vi "Read Data.vi"(8 "error in (no error)":errorcluster, 11 "VISA resource name":refnum<visa-resource-name>) -> (0 "error out":errorcluster, 1 "Return String":string, 2 "Data Value":dbl format="%_10f", 3 "VISA resource name out":refnum<visa-resource-name>)   [LabVIEW 2019, in "BK Precision 1823A.lvlib"]
doc: "This VI returns the measured data corresponding to the display of the counter."
uses:
  BK Precision 1823A.lvlib
panel:
  # "Units"
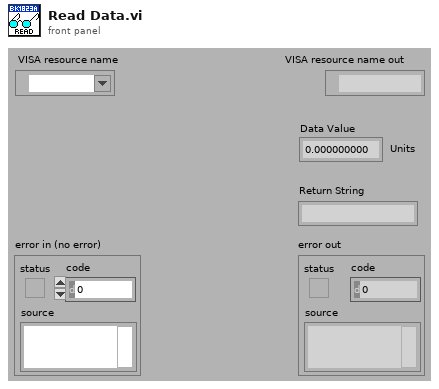
[diagram p1: front panel]
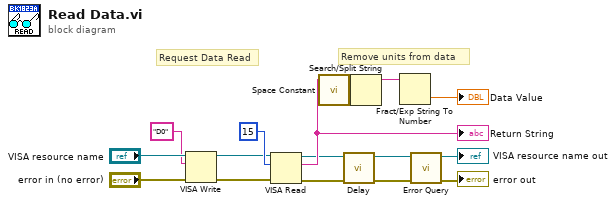
[diagram p0: block diagram]
diagram:
  # "Remove units from data"
  # "Request Data Read"
  n1 = VISA Write(VISA resource name="VISA resource name", write buffer="D0", error in (no error)="error in (no error)") -> (VISA resource name out=w12:refnum<visa-resource-name>, error out=w11:errorcluster)  [unwired: 1 out]
  n2 = VISA Read(VISA resource name=w12, byte count=15, error in (no error)=w11) -> (VISA resource name out=w1:refnum<visa-resource-name>, read buffer=w8:string, error out=w4:errorcluster)  [unwired: 1 out]
  "Return String" <- w8
  n3 = call <vilib>:"Space Constant.vi"() -> ("String"=w7:string)
  n4 = call "Delay.vi"("error in (no error)"=w4, "VISA resource name"=w1) -> ("error out"=w3:errorcluster, "VISA resource name out"=w2:refnum<visa-resource-name>)  [unwired: 8 in]
  n5 = Search/Split String(string=w8, search string/char (-)=w7) -> (substring before match=w6:string)  [unwired: 1 in, 2 out]
  n6 = Fract/Exp String To Number(string=w6) -> (number=→"Data Value":dbl)  [unwired: 3 in, 1 out]
  n7 = call "Error Query.vi"("error in (no error)"=w3, "VISA resource name"=w2) -> ("error out"=→"error out":errorcluster, "VISA resource name out"=→"VISA resource name out":refnum<visa-resource-name>)  [unwired: 8 in]
